vi "ClearSubPanelStandardEvents.vi"(8 "error in":errorcluster, 10 "standard events":T1, 11 "sub panel ref in":refnum<vi>) -> (0 "error out":errorcluster, 3 "sub panel ref out":refnum<vi>)   [LabVIEW 2013, in "NISE_CEF_TreeControl.lvlib"]
uses:
  NISE_CEF_TreeControl.lvlib
  Node/StandardEvents.ctl
  Node/UserEventRef.ctl
  Controls/EventCluster.ctl
  Node/NodeChangeEvent.ctl
  Node/NodeRef.ctl
  Node/NISE_CEF_Node.lvclass
  Node/CacheState.ctl
  Node/RefreshUIEvent.ctl
  Node/StopEvent.ctl
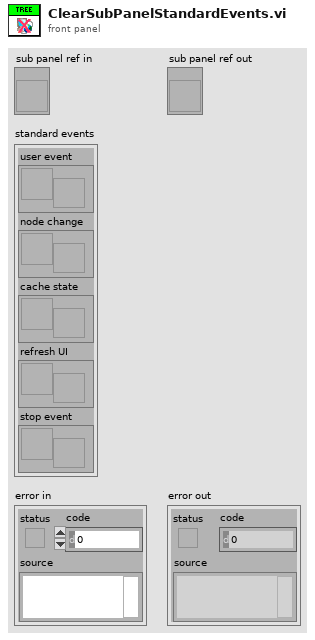
[diagram p1: front panel]
types:
  T1 = typedef "NISE_CEF_Node.lvclass/StandardEvents.ctl" = cluster{"user event":T2, "node change":T3, "cache state":T4, "refresh UI":T5, "stop event":T6}
  T2 = typedef "NISE_CEF_Node.lvclass/UserEventRef.ctl" = refnum<user-event>
  T3 = typedef "NISE_CEF_Node.lvclass/NodeChangeEvent.ctl" = refnum<user-event>
  T4 = typedef "NISE_CEF_Node.lvclass/CacheState.ctl" = refnum<user-event>
  T5 = typedef "NISE_CEF_Node.lvclass/RefreshUIEvent.ctl" = refnum<user-event>
  T6 = typedef "NISE_CEF_Node.lvclass/StopEvent.ctl" = refnum<user-event>
  T7 = typedef "NISE_CEF_TreeControl.lvlib/EventCluster.ctl" = cluster{"command":string, "data":string}
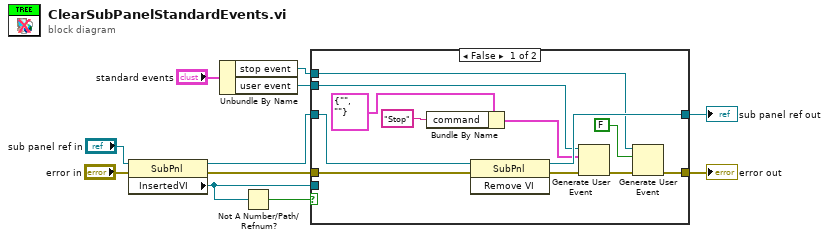
[diagram p0: block diagram]
diagram:
  n1 = property class="SubPnl"(reference="sub panel ref in", error in="error in") -> (reference out=w11:refnum<vi>, error out=w9:errorcluster, "InsertedVI"=w7:refnum<vi>)
  n2 = Unbundle By Name("standard events") -> ("stop event"=w1:T6, "user event"=w2:T2)
  n3 = Not A Number/Path/Refnum?(number/path/refnum=w7) -> (NaN/Path/Refnum?=w10:bool)
  n4 = case shown="False" w10 {
    tunnel: [w14 w25] -> w4
    tunnel: w7 -> [_ _]
    tunnel: w11 -> [w23 w24]
    tunnel: w9 -> [w20 w25]
    tunnel: [w22 w24] -> w5
    tunnel: w2 -> [w21 _]
    tunnel: w1 -> [w13 _]
    frame False {
      n5 = Bundle By Name(cluster=T7 {"command"="", "data"=""} ("event data"), "command"="Stop") -> (w16:T7)
      n6 = invoke class="SubPnl" method="Remove VI"(reference=w23, error in=w20) -> (reference out=w22:refnum<vi>, error out=w19:errorcluster)  [unwired: 1 in, 1 out]
      n7 = Generate User Event(user event=w21, event data cluster=w16, error in=w19) -> (error out=w18:errorcluster)  [unwired: 1 in, 1 out]
      n8 = Generate User Event(user event=w13, event data cluster=FALSE ("event data"), error in=w18) -> (error out=w14:errorcluster)  [unwired: 1 in, 1 out]
    }
    frame True {
      # "Reference is not valid if there is no VI"
    }
  }
  "error out" <- w4
  "sub panel ref out" <- w5
